vi "Monitor DTCs.vi"(8 "error in":errorcluster, 11 "J1939 internal data":T1={"J1939 XNET Settings"={"XNET Database"="", "XNET Cluster"="", "CAN port"="", "Baud rate [Bd]"=0, "J1939 Network Address"=0, "Name"=0, "Termination"=0}, "j1939 queues"={"Processed Outgoing"=refnum, "Process Outgoing"=refnum, "stop notifier"=refnum, "error queue"=refnum, "active dtc"=refnum, "processed inc"=refnum}, "fgv references"={"BAM Buffer"=refnum, "CM Buffer"=refnum, "CM Gen"=refnum, "BAM Gen"=refnum, "Address Claims"=refnum, "RQST"=refnum, "scaling lut"=refnum, "data lut"=refnum, "cyclic scheduler"=refnum}, "frame in"="", "frame out"="", "timing"={"tb to j1939 queue timeout"=100, "j1939 to tb queue timeout"=100, "dtc loop period (ms)"=100, "CAN in loop period (ms)"=100, "process incoming queue timeout (ms)"=100, "Outgoing Write Decimation"=0, "process outgoing loop rate (ms)"=0, "periodic outgoing queue timeout (ms)"=10, "CAN out queue timeout (ms)"=100}}) -> ()   [LabVIEW 2013, in "J1939.lvlib"]
uses:
  J1939.lvlib
  API Types/Internal Data.ctl
  API Types/XNET Settings.ctl
  API Types/Setup Information Cluster.ctl
  API Types/CAN Outgoing Message Cluster.ctl
  API Types/Convert DTCs Cluster.ctl
  <vilib>/xnet/xnet.llb/XNET Frame CAN.ctl
  <vilib>/xnet/xnet.llb/XNET Frame Type CAN.ctl
  TP/TP List References.ctl
  BAM/BAM Buffer Connections List_Ref.ctl
  Connection Mode/Connection Mode Generation Connection Ref.ctl
  BAM/BAM Generation Connections List_Ref.ctl
  LUTs/J1939 Address Table Reference.ctl
  RQST/RQST Lookup Table Reference.ctl
  LUTs/J1939 Conversion Lookup Table Reference.ctl
  LUTs/J1939 Data Lookup Table Reference.ctl
  LUTs/Cyclic Frame Scheduler Lut Reference.ctl
  Configuration/TypeDefs/timing configuration.ctl
  CD/CD Address Lookup Table.vi
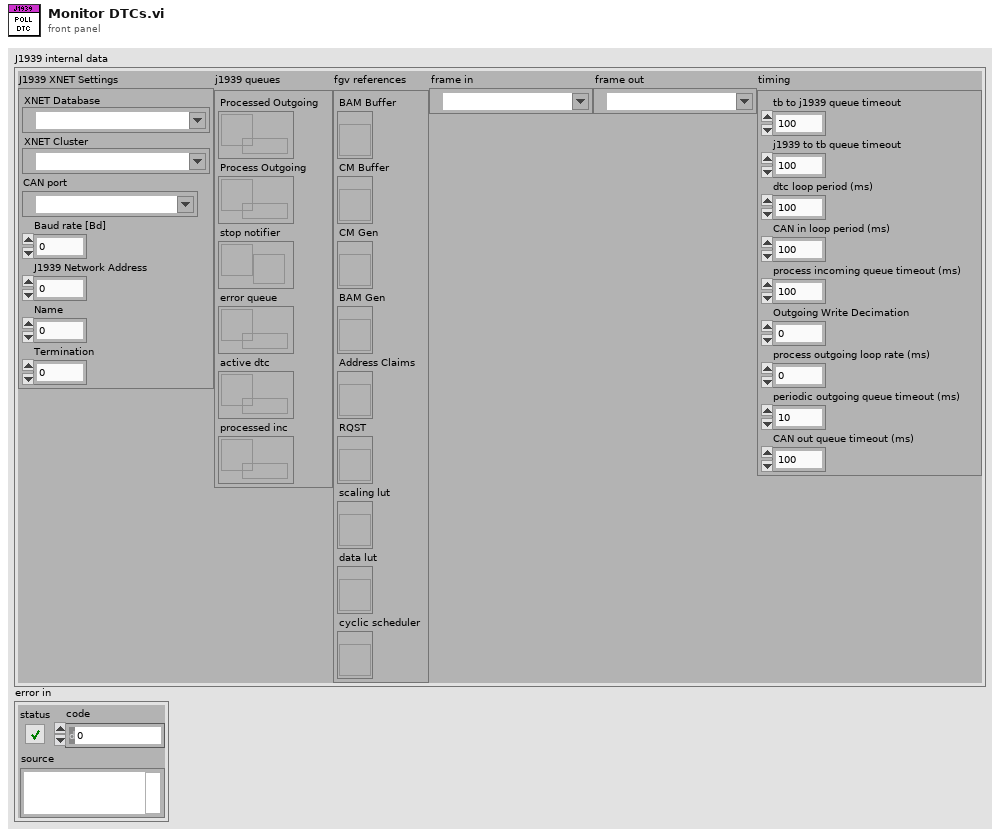
[diagram p1: front panel]
types:
  T1 = typedef "J1939.lvlib/Internal Data.ctl" = cluster{"J1939 XNET Settings":T2, "j1939 queues":T3, "fgv references":T4, "frame in":refnum<k21>, "frame out":refnum<k21>, "timing":T13}
  T2 = typedef "J1939.lvlib/XNET settings.ctl" = cluster{"XNET Database":refnum<k21>, "XNET Cluster":refnum<k21>, "CAN port":refnum<k21>, "Baud rate [Bd]":u32, "J1939 Network Address":u8, "Name":u64, "Termination":u32}
  T3 = typedef "J1939.lvlib/Setup Information Cluster.ctl" = cluster{"Processed Outgoing":refnum<queue>, "Process Outgoing":refnum<queue>, "stop notifier":refnum<notifier>, "error queue":refnum<queue>, "active dtc":refnum<queue>, "processed inc":refnum<queue>}
  T4 = typedef "J1939.lvlib/TP List References.ctl" = cluster{"BAM Buffer":T5, "CM Buffer":T5, "CM Gen":T6, "BAM Gen":T7, "Address Claims":T8, "RQST":T9, "scaling lut":T10, "data lut":T11, "cyclic scheduler":T12}
  T5 = typedef "J1939.lvlib/BAM Buffer Connections List_Ref.ctl" = refnum<vi>
  T6 = typedef "J1939.lvlib/Connection Mode Generation Connection Ref.ctl" = refnum<vi>
  T7 = typedef "J1939.lvlib/BAM Generation Connections List_Ref.ctl" = refnum<vi>
  T8 = typedef "J1939.lvlib/J1939 Address Table Reference.ctl" = refnum<vi>
  T9 = typedef "J1939.lvlib/RQST Lookup Table Reference.ctl" = refnum<vi>
  T10 = typedef "J1939.lvlib/J1939 Conversion Lookup Table Reference.ctl" = refnum<vi>
  T11 = typedef "J1939.lvlib/J1939 Data Lookup Table Reference.ctl" = refnum<vi>
  T12 = typedef "J1939.lvlib/cyclic frame scheduler lut reference.ctl" = refnum<vi>
  T13 = typedef "J1939.lvlib/timing configuration.ctl" = cluster{"tb to j1939 queue timeout":i32, "j1939 to tb queue timeout":i32, "dtc loop period (ms)":i32, "CAN in loop period (ms)":i32, "process incoming queue timeout (ms)":i32, "Outgoing Write Decimation":u32, "process outgoing loop rate (ms)":i32, "periodic outgoing queue timeout (ms)":i32, "CAN out queue timeout (ms)":i32}
  T14 = typedef "J1939.lvlib/J1939 Address Lookup Table Data.ctl" = cluster{"Name":u8[], "Address":u8}
  T15 = typedef "J1939.lvlib/Convert DTCs Cluster.ctl" = cluster{"Lamps":cluster{"Malfunction Indicator":u8, "Red Stop":u8, "Amber Warning":u8, "Protect Lamp":u8}, "DTCs":cluster{"SPN":u32, "FMI":u8, "Occurrance":u8}[], "Active?":bool, "Address":u8, "timestamp":timestamp}
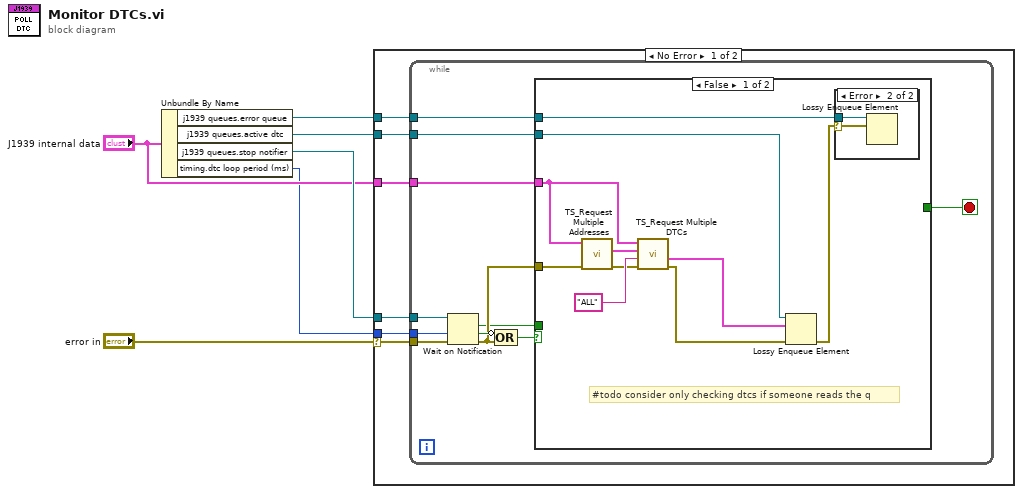
[diagram p0: block diagram]
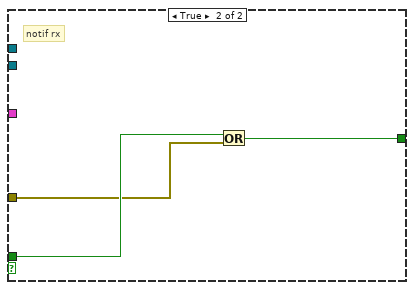
[diagram p3: hidden frame]
diagram:
  n1 = Unbundle By Name("J1939 internal data") -> ("j1939 queues.error queue"=w5:refnum<queue>, "j1939 queues.active dtc"=w2:refnum<queue>, "j1939 queues.stop notifier"=w6:refnum<notifier>, "timing.dtc loop period (ms)"=w1:i32)
  n2 = case shown="No Error" "error in" {
    selector: "error in" -> [w12 _]
    tunnel: w6 -> [w11 _]
    tunnel: w1 -> [w10 _]
    tunnel: "J1939 internal data" -> [w9 _]
    tunnel: w5 -> [w8 _]
    tunnel: w2 -> [w7 _]
    frame No Error {
      n3 = while {
        tunnel: w11 -> [w22]
        tunnel: w12 -> [w23]
        tunnel: w10 -> [w16]
        tunnel: w9 -> [w15]
        tunnel: w8 -> [w14]
        tunnel: w7 -> [w13]
        stop <- w17 stop-if-true
        n4 = Wait on Notification(notifier=w22, timeout in ms (-1)=w16, error in (no error)=w23) -> (notification=w18:bool, timed out?=w21:bool, error out=w19:errorcluster)  [unwired: 1 in, 1 out]
        n5 = Compound Arithmetic op=OR(invert w21, w19) -> (w20:bool)
        n6 = case shown="False" w20 {
          tunnel: w19 -> [w29 w36]
          tunnel: w18 -> [_ w38]
          tunnel: [_ w37] -> w17
          tunnel: w15 -> [w28 _]
          tunnel: w14 -> [w33 _]
          tunnel: w13 -> [w25 _]
          frame False {
            # "#todo consider only checking dtcs if someone reads the q"
            n7 = call "TS_Request Multiple Addresses.vi"("error in"=w29, "internal data"=w28) -> ("error out"=w30:errorcluster, "addresses"=w31:T14[])  [unwired: 8 in]
            n8 = call "TS_Request Multiple DTCs.vi"("error in"=w30, "Command"="ALL", "addresses"=w31, "internal data"=w28) -> ("error out"=w27:errorcluster, "Responses"=w26:T15[])  [unwired: 6 in]
            n9 = Lossy Enqueue Element(queue=w25, element=w26, error in (no error)=w27) -> (error out=w24:errorcluster)  [unwired: 3 out]
            n10 = case shown="Error" w24 {
              selector: w24 -> [_ w35]
              tunnel: w33 -> [_ w34]
              frame No Error {
              }
              frame Error {
                n11 = Lossy Enqueue Element(queue=w34, element=w35) -> ()  [unwired: 1 in, 4 out]
              }
            }
          }
          frame True {
            # "notif rx"
            n12 = Or(x=w38, y=w36) -> (x .or. y?=w37:bool)
          }
        }
      }
    }
    frame Error {
    }
  }
